vi "BuildBandPlot2.vi"(10 "Data In":T2(graph), 11 "CrsrList":T1) -> (2 "Normalized FFT":T3(graph), 3 "Array":dbl[](array[numeric]))   [LabVIEW 2014]
uses:
  <vilib>/Utility/miscctls.llb/LVCursorListTypeDef.ctl
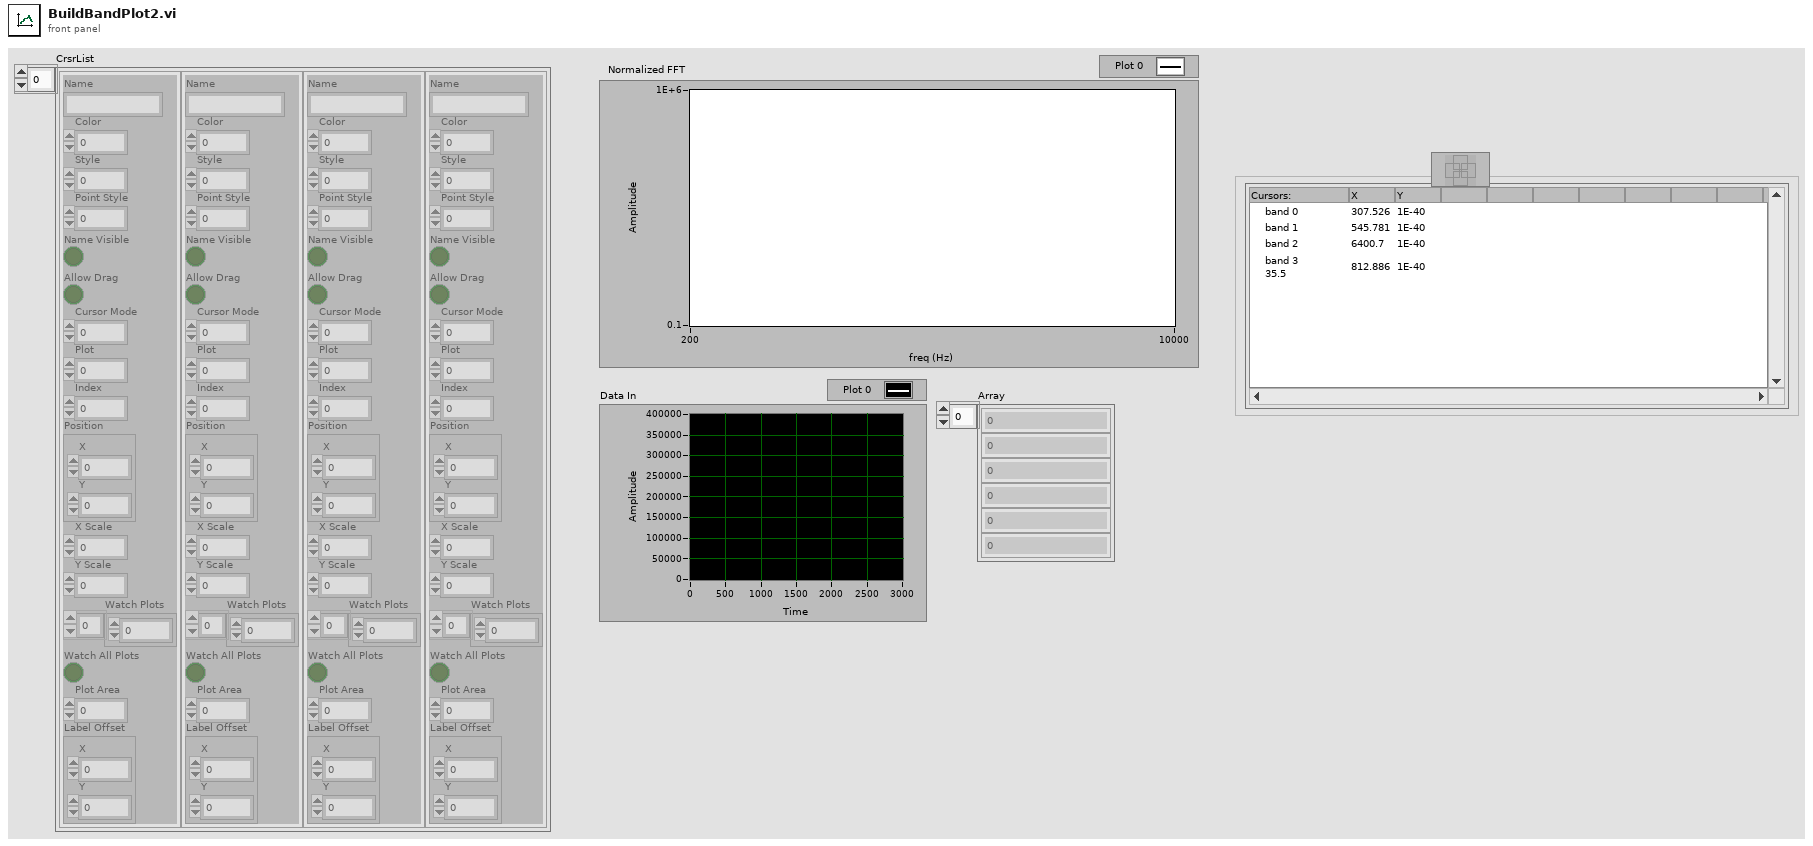
[diagram p1: front panel]
types:
  T1 = typedef "LVCursorListTypeDef.ctl" = cluster{"Name":string, "Color":u32, "Style":u8, "Point Style":u8, "Name Visible":bool, "Allow Drag":bool, "Cursor Mode":u32, "Plot":i32, "Index":i32, "Position":cluster{"X":dbl, "Y":dbl}, "X Scale":u32, "Y Scale":u32, "Watch Plots":i32[], "Watch All Plots":bool, "Plot Area":i32, "Label Offset":cluster{"X":dbl, "Y":dbl}}[]
  T2 = cluster{dbl, "df":dbl, "Power Spectrum (V^2 rms)":dbl[]}
  T3 = cluster{dbl, "df":dbl, "Power Spectrum (V^2 rms)":dbl[]}[]
  T4 = cluster{"X":dbl, cluster{"Name":string, "Color":u32, "Style":u8, "Point Style":u8, "Name Visible":bool, "Allow Drag":bool, "Cursor Mode":u32, "Plot":i32, "Index":i32, "Position":cluster{"X":dbl, "Y":dbl}, "X Scale":u32, "Y Scale":u32, "Watch Plots":i32[], "Watch All Plots":bool, "Plot Area":i32, "Label Offset":cluster{"X":dbl, "Y":dbl}}}
  T5 = cluster{"X":dbl, cluster{"Name":string, "Color":u32, "Style":u8, "Point Style":u8, "Name Visible":bool, "Allow Drag":bool, "Cursor Mode":u32, "Plot":i32, "Index":i32, "Position":cluster{"X":dbl, "Y":dbl}, "X Scale":u32, "Y Scale":u32, "Watch Plots":i32[], "Watch All Plots":bool, "Plot Area":i32, "Label Offset":cluster{"X":dbl, "Y":dbl}}}[]
  T6 = cluster{"Name":string, "Color":u32, "Style":u8, "Point Style":u8, "Name Visible":bool, "Allow Drag":bool, "Cursor Mode":u32, "Plot":i32, "Index":i32, "Position":cluster{"X":dbl, "Y":dbl}, "X Scale":u32, "Y Scale":u32, "Watch Plots":i32[], "Watch All Plots":bool, "Plot Area":i32, "Label Offset":cluster{"X":dbl, "Y":dbl}}
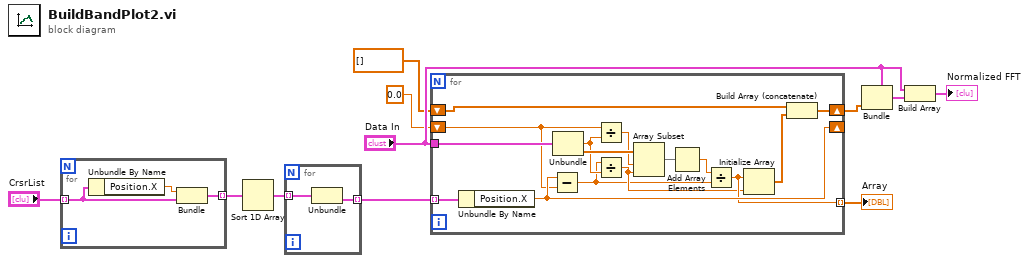
[diagram p0: block diagram]
diagram:
  n1 = for {
    tunnel: "CrsrList" -> [w13] mode=indexing
    tunnel: [w12] -> w4 mode=indexing
    n2 = Unbundle By Name(w13) -> ("Position.X"=w14:dbl)
    n3 = Bundle("X"=w14, w13) -> (w12:T4)  [unwired: 1 in]
  }
  n4 = Sort 1D Array(array=w4) -> (sorted array=w3:T5)
  n5 = for {
    tunnel: w3 -> [w16] mode=indexing
    tunnel: [w15] -> w1 mode=indexing
    n6 = Unbundle(w16) -> (w15:T6)  [unwired: 1 out]
  }
  n7 = for {
    tunnel: w1 -> [w31] mode=indexing
    tunnel: "Data In" -> [w30]
    shift-right: [w24] -> _
    shift-left: 0.0 -> [w23]
    tunnel: [w22] -> w6 mode=indexing
    shift-right: [w18] -> w8
    shift-left: dbl[] [] -> [w20]
    n8 = Unbundle By Name(w31) -> ("Position.X"=w24:dbl)
    n9 = Subtract(x=w24, y=w23) -> (x-y=w17:dbl)
    n10 = Unbundle(w30) -> ("df"=w26:dbl, "Power Spectrum (V^2 rms)"=w29:dbl[])  [unwired: 1 out]
    n11 = Divide(x=w23, y=w26) -> (x/y=w25:dbl)
    n12 = Divide(x=w17, y=w26) -> (x/y=w21:dbl)
    n13 = Array Subset(array=w29, index=w25, length=w21) -> (w28:dbl[])
    n14 = Add Array Elements(numeric array=w28) -> (sum=w27:dbl)
    n15 = Divide(x=w27, y=w17) -> (x/y=w22:dbl)
    n16 = Initialize Array(w22, w21) -> (w19:dbl[])
    n17 = Build Array (concatenate)(w20, w19) -> (w18:dbl[])
  }
  "Array" <- w6
  n18 = Bundle(cluster="Data In", "Power Spectrum (V^2 rms)"=w8) -> (w9:T2)  [unwired: 2 in]
  n19 = Build Array("Data In", w9) -> (→"Normalized FFT":T3)
